vi "subSetupSubDlg.vi"(1 "viref subdlg":refnum<vi>, 2 "Reference":T1) -> (0 "subDlgRefs":refnum<vi>[](array[refnum]))   [LabVIEW 2020]
uses:
  <vilib>/express/express shared/propPageData.ctl
panel:
  out "Array 3":variant[](array[variant])
  out "Array 2":string[](array[string])
  out "Array":bool[](array[boolean])
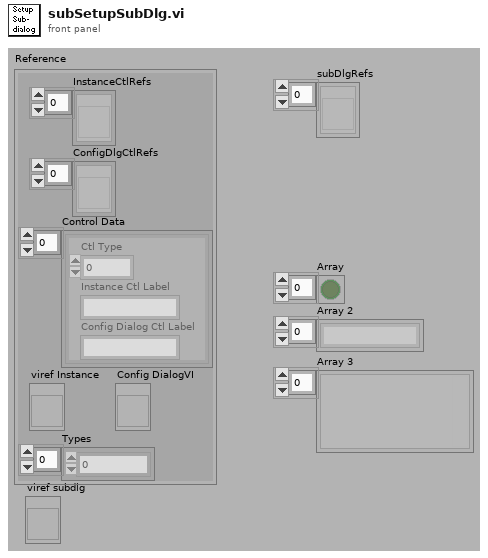
[diagram p1: front panel]
types:
  T1 = typedef "propPageData.ctl" = cluster{"InstanceCtlRefs":refnum<vi>[], "ConfigDlgCtlRefs":refnum<vi>[], "Control Data":cluster{"Ctl Type":u16, "Instance Ctl Label":string, "Config Dialog Ctl Label":string}[], "viref Instance":refnum<vi>, "Types":i32[], "Config DialogVI":refnum<vi>}
  T2 = cluster{"Ctl Type":u16, "Instance Ctl Label":string, "Config Dialog Ctl Label":string}[]
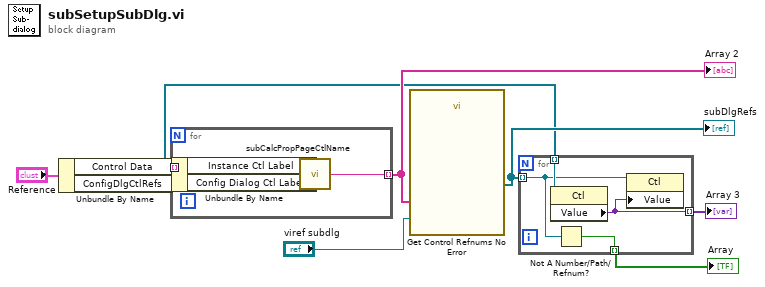
[diagram p0: block diagram]
diagram:
  n1 = Unbundle By Name("Reference") -> ("Control Data"=w8:T2, "ConfigDlgCtlRefs"=w5:refnum<vi>[])
  n2 = for {
    tunnel: w8 -> [w12] mode=indexing
    tunnel: [w9] -> w7 mode=indexing
    n3 = Unbundle By Name(w12) -> ("Instance Ctl Label"=w11:string, "Config Dialog Ctl Label"=w10:string)
    n4 = call <vilib>:"subCalcPropPageCtlName.vi"("Property Page Ctl Label"=w10, "Express VI Ctl Label"=w11) -> ("Prop Ctl Name"=w9:string)
  }
  "Array 2" <- w7
  n5 = call <vilib>:"Get Control Refnums No Error.vi"("Names"=w7, "viref Block"="viref subdlg") -> ("Refs Output"=w6:refnum<vi>[])  [unwired: 2 in, 7 out]
  "subDlgRefs" <- w6
  n6 = for {
    tunnel: w6 -> [w14] mode=indexing
    tunnel: w5 -> [w15] mode=indexing
    tunnel: [w13] -> w4 mode=indexing
    tunnel: [w16] -> w2 mode=indexing
    n7 = property class="Ctl"(reference=w15) -> ("Value"=w16:variant)  [unwired: 1 in, 2 out]
    n8 = Not A Number/Path/Refnum?(number/path/refnum=w14) -> (NaN/Path/Refnum?=w13:bool)
    n9 = property class="Ctl"(reference=w14, "Value"=w16) -> ()  [unwired: 1 in, 2 out]
  }
  "Array" <- w4
  "Array 3" <- w2
